vi "Area_Triangulo.vi"() -> ()   [LabVIEW 2020]
panel:
  out "Perimetro":dbl
  out "Area":dbl
  in  "Altura":dbl
  in  "Base":dbl
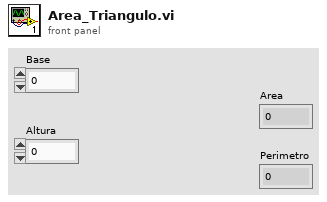
[diagram p1: front panel]
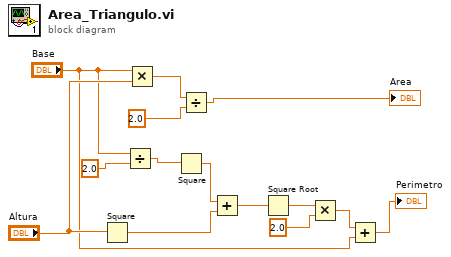
[diagram p0: block diagram]
diagram:
  n1 = Square(x="Altura") -> (x^2=w9:dbl)
  n2 = Divide(x="Base", y=2.0) -> (x/y=w12:dbl)
  n3 = Multiply(x="Base", y="Altura") -> (x*y=w14:dbl)
  n4 = Square(x=w12) -> (x^2=w10:dbl)
  n5 = Divide(x=w14, y=2.0) -> (x/y=→"Area":dbl)
  n6 = Add(x=w10, y=w9) -> (x+y=w8:dbl)
  n7 = Square Root(x=w8) -> (sqrt(x)=w7:dbl)
  n8 = Multiply(x=w7, y=2.0) -> (x*y=w6:dbl)
  n9 = Add(x=w6, y="Base") -> (x+y=→"Perimetro":dbl)
